vi "ParseObjectXML.vi"(8 "error in (no error)":errorcluster, 11 "Object XML":string="  <Object>\n    <Name>Blah</Name>\n    <Class>CoilQF_Test</Class>\n    <Config>\n      <NumElts>1</NumElts>\n      <String>\n        <Name>Rig_Location</Name>\n        <Val>Sydney</Val>\n      </String>\n    </Config>\n    <Validation>\n      <Method>\n        <Name>GetVersion</Name>\n        <Value>V1.2</Value>\n      </Method>\n      <Method>\n        <Name>GetCallChain</Name>\n        <Value>ViKingBase:Blah</Value>\n      </Method>\n    </Validation>\n    <Objects>\n          <Object>\n            <Name>Crud</Name>\n            <Class>Crud_class</Class>\n          </Object>\n      <Object>\n        <Name>QFM</Name>\n        <Class>QFM_T457232</Class>\n        <Config>\n          <NumElts>1</NumElts>\n          <String>\n            <Name>COM_Port</Name>\n            <Val>COM4</Val>\n          </String>\n        </Config>\n        <Validation>\n          <Method>\n            <Name>GetModel</Name>\n            <Value>T457635</Value>\n          </Method>\n          <Method>\n            <Name>GetSN</Name>\n            <Value>12</Value>\n          </Method>\n        </Validation>\n      </Object>\n    </Objects>\n    <Ancestors>\n      <Ancestor>\n        <Class>ViKing_Test_Base</Class>\n        <Config>\n          <NumElts>1</NumElts>\n          <String>\n            <Name>Rig_Location</Name>\n            <Val>Sydney</Val>\n          </String>\n        </Config>\n        <Objects>\n          <Object>\n            <Name>TestView</Name>\n            <Class>TestView_Tree</Class>\n          </Object>\n          <Object>\n            <Name>Crud</Name>\n            <Class>Crud_class</Class>\n          </Object>\n        </Objects>\n      </Ancestor>\n    </Ancestors>\n  </Object>") -> (0 "error out":errorcluster, 3 "Object Cluster":T1)   [LabVIEW 2022 SP3, in "ViPER.lvlib" / "ViPER.lvclass"]
doc: "### BSD License (http://www.opensource.org/licenses/bsd-license.php) Begin ###\n\nCopyright (c) 2018 Kurt Friday www.medulla.net\n\nAll rights reserved.\n\nRedistribution and use in source and binary forms, with or without\nmodification, are permitted provided that the following conditions are met:\n\n * Redistributions of source code must retain the above copyright\n notice, this list of conditions and the following disclaimer.\n\n * Redistributions in binary form must reproduce the above copyright\n notice, this list of conditions and the following disclaimer in the\n documentation and/or other materials provided with the distribution.\n\n * Neither the name of the <organization> nor the\n names of its contributors may be used to endorse or promote products\n derived from this software without specific prior written permission.\n\nTHIS SOFTWARE IS PROVIDED BY THE COPYRIGHT HOLDERS AND CONTRIBUTORS \"AS IS\" AND\nANY EXPRESS OR IMPLIED WARRANTIES, INCLUDING, BUT NOT LIMITED TO, THE IMPLIED\nWARRANTIES OF MERCHANTABILITY AND FITNESS FOR A PARTICULAR PURPOSE ARE\nDISCLAIMED. IN NO EVENT SHALL <COPYRIGHT HOLDER> BE LIABLE FOR ANY\nDIRECT, INDIRECT, INCIDENTAL, SPECIAL, EXEMPLARY, OR CONSEQUENTIAL DAMAGES\n(INCLUDING, BUT NOT LIMITED TO, PROCUREMENT OF SUBSTITUTE GOODS OR SERVICES;\nLOSS OF USE, DATA, OR PROFITS; OR BUSINESS INTERRUPTION) HOWEVER CAUSED AND\nON ANY THEORY OF LIABILITY, WHETHER IN CONTRACT, STRICT LIABILITY, OR TORT\n(INCLUDING NEGLIGENCE OR OTHERWISE) ARISING IN ANY WAY OUT OF THE USE OF THIS\nSOFTWARE, EVEN IF ADVISED OF THE POSSIBILITY OF SUCH DAMAGE."
uses:
  ViPER.lvclass
  ObjectDefinition.ctl
  Ancestor.ctl
  <vilib>/xml/Load XML String.vi
  <vilib>/xml/Close Reference(Node).vi
  <vilib>/xml/NI_XML.lvlib
panel:
  # "### BSD License (http://www.opensource.org/licenses/bsd-license.php) Begin ###\n\nCopyright (c) 2018  Kurt Friday www.medulla.net\n\nAll rights reserved.\n\nRedistribution and use in source and binary forms, with or without\nmodification, are permitted provided that the following conditions are met:\n\n    * Redistributions of source code must retain the above copyright\n      notice, this list of conditions and the following disclaimer.\n\n    * Redistributions in binary form must reproduce the above copyright\n      notice, this list of conditions and the following disclaimer in the\n      documentation and/or other materials provided with the distribution.\n\n    * Neither the name of the <organization> nor the\n      names of its contributors may be used to endorse or promote products\n      derived from this software without specific prior written permission.\n\nTHIS SOFTWARE IS PROVIDED BY THE COPYRIGHT HOLDERS AND CONTRIBUTORS \"AS IS\" AND\nANY EXPRESS OR IMPLIED WARRANTIES, INCLUDING, BUT NOT LIMITED TO, THE IMPLIED\nWARRANTIES OF MERCHANTABILITY AND FITNESS FOR A PARTICULAR PURPOSE ARE\nDISCLAIMED. IN NO EVENT SHALL <COPYRIGHT HOLDER> BE LIABLE FOR ANY\nDIRECT, INDIRECT, INCIDENTAL, SPECIAL, EXEMPLARY, OR CONSEQUENTIAL DAMAGES\n(INCLUDING, BUT NOT LIMITED TO, PROCUREMENT OF SUBSTITUTE GOODS OR SERVICES;\nLOSS OF USE, DATA, OR PROFITS; OR BUSINESS INTERRUPTION) HOWEVER CAUSED AND\nON ANY THEORY OF LIABILITY, WHETHER IN CONTRACT, STRICT LIABILITY, OR TORT\n(INCLUDING NEGLIGENCE OR OTHERWISE) ARISING IN ANY WAY OUT OF THE USE OF THIS\nSOFTWARE, EVEN IF ADVISED OF THE POSSIBILITY OF SUCH DAMAGE."
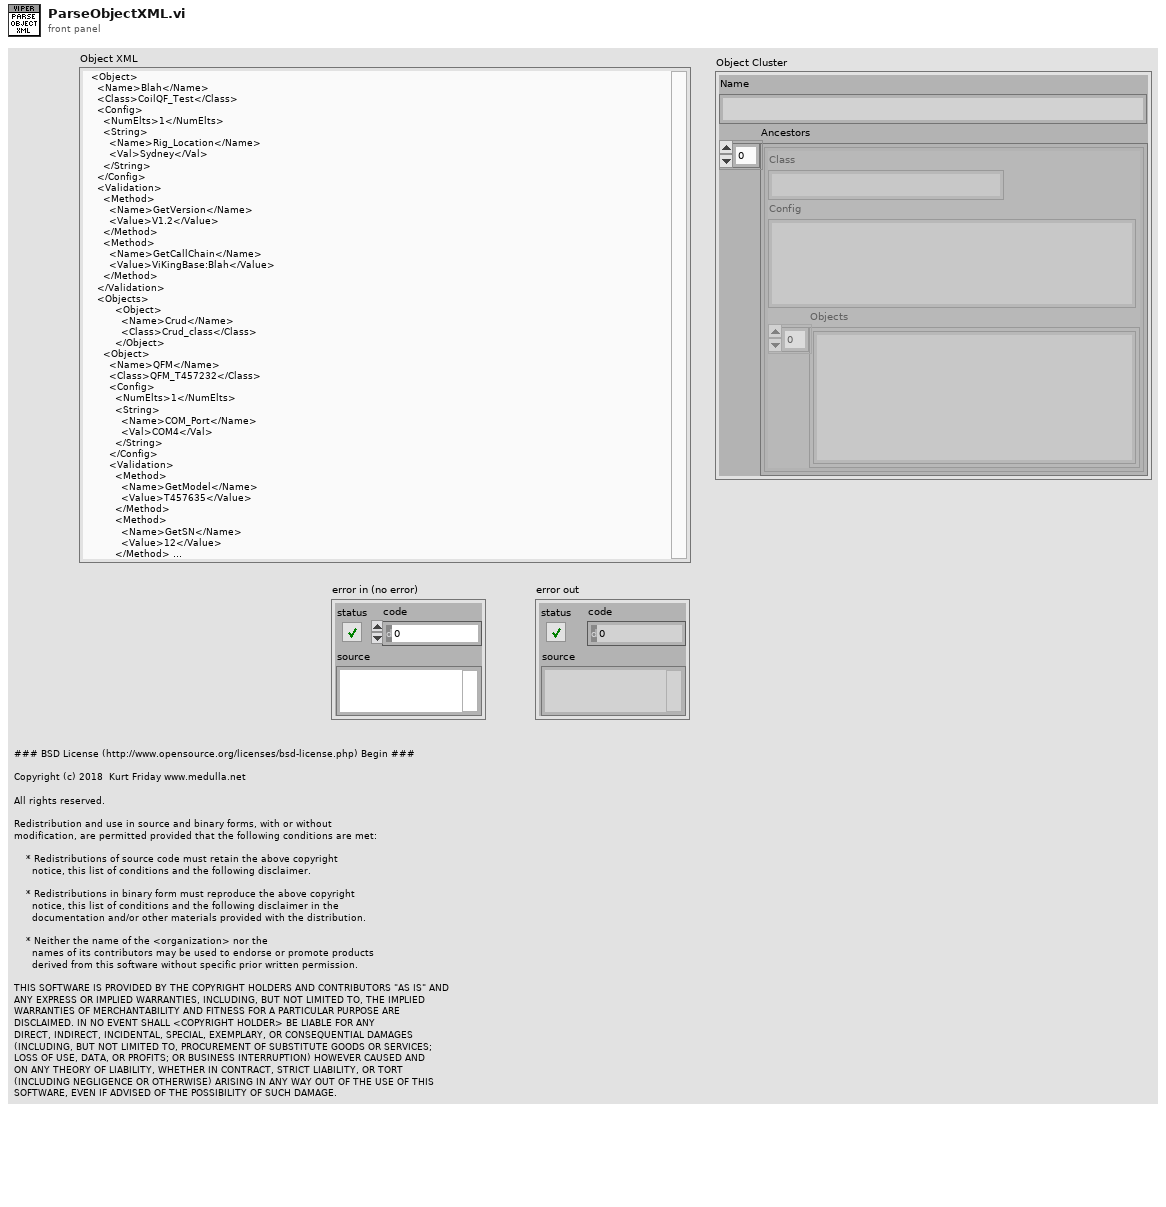
[diagram p1: front panel]
types:
  T1 = typedef "ViPER.lvlib/ViPER.lvclass/ObjectDefinition.ctl" = cluster{"Name":string, "Ancestors":T2[]}
  T2 = typedef "ViPER.lvlib/ViPER.lvclass/Ancestor.ctl" = cluster{"Class":string, "Config":string, "Objects":string[]}
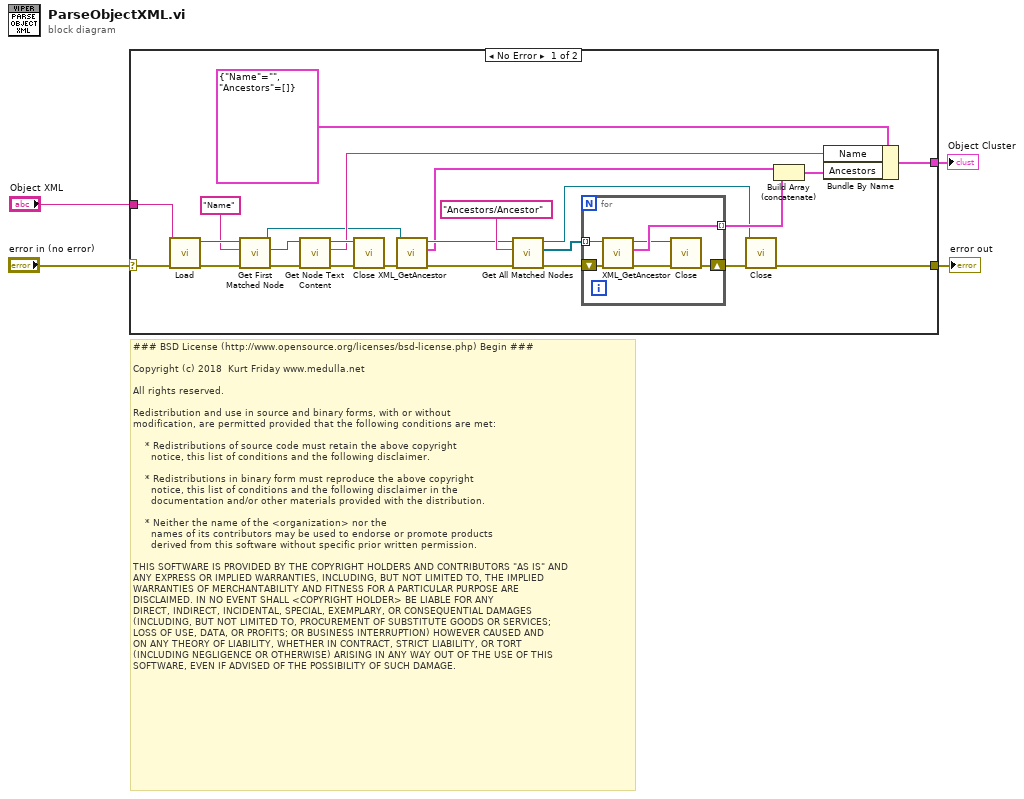
[diagram p0: block diagram]
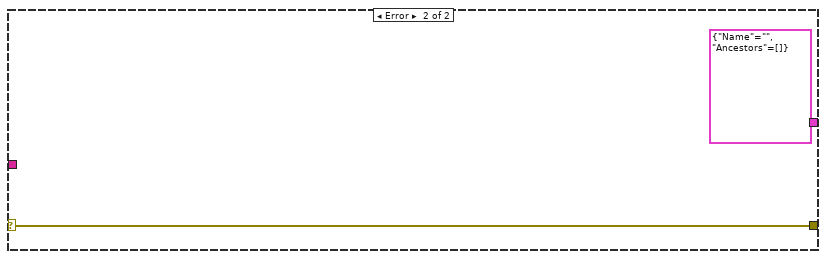
[diagram p2: hidden frame]
diagram:
  # "### BSD License (http://www.opensource.org/licenses/bsd-license.php) Begin ###\n\nCopyright (c) 2018  Kurt Friday www.medulla.net\n\nAll rights reserved.\n\nRedistribution and use in source and binary forms, with or without\nmodification, are permitted provided that the following conditions are met:\n\n    * Redistributions of source code must retain the above copyright\n      notice, this list of conditions and the following disclaimer.\n\n    * Redistributions in binary form must reproduce the above copyright\n      notice, this list of conditions and the following disclaimer in the\n      documentation and/or other materials provided with the distribution.\n\n    * Neither the name of the <organization> nor the\n      names of its contributors may be used to endorse or promote products\n      derived from this software without specific prior written permission.\n\nTHIS SOFTWARE IS PROVIDED BY THE COPYRIGHT HOLDERS AND CONTRIBUTORS \"AS IS\" AND\nANY EXPRESS OR IMPLIED WARRANTIES, INCLUDING, BUT NOT LIMITED TO, THE IMPLIED\nWARRANTIES OF MERCHANTABILITY AND FITNESS FOR A PARTICULAR PURPOSE ARE\nDISCLAIMED. IN NO EVENT SHALL <COPYRIGHT HOLDER> BE LIABLE FOR ANY\nDIRECT, INDIRECT, INCIDENTAL, SPECIAL, EXEMPLARY, OR CONSEQUENTIAL DAMAGES\n(INCLUDING, BUT NOT LIMITED TO, PROCUREMENT OF SUBSTITUTE GOODS OR SERVICES;\nLOSS OF USE, DATA, OR PROFITS; OR BUSINESS INTERRUPTION) HOWEVER CAUSED AND\nON ANY THEORY OF LIABILITY, WHETHER IN CONTRACT, STRICT LIABILITY, OR TORT\n(INCLUDING NEGLIGENCE OR OTHERWISE) ARISING IN ANY WAY OUT OF THE USE OF THIS\nSOFTWARE, EVEN IF ADVISED OF THE POSSIBILITY OF SUCH DAMAGE."
  n1 = case shown="No Error" "error in (no error)" {
    selector: "error in (no error)" -> [w5 w37]
    tunnel: "Object XML" -> [w28 _]
    tunnel: [w7 T1 {"Name"="", "Ancestors"=[]} ("Object")] -> w3
    tunnel: [w6 w37] -> w2
    frame No Error {
      n2 = call-poly <vilib>:"Load.vi"("XML string"=w28, "error in (no error)"=w5) -> ("DOM document out"=w27:refnum<k20>, "error out"=w29:errorcluster)  [unwired: 11 in, 1 out]
      n3 = call <vilib>:"Get First Matched Node.vi"("error in (no error)"=w29, "XPath expression"="Name", "node in"=w27) -> ("error out"=w24:errorcluster, "node result"=w21:refnum<k20>, "node out"=w18:refnum<k20>)  [unwired: 6 in]
      n4 = call <vilib>:"Get Node Text Content.vi"("error in (no error)"=w24, "node in"=w21) -> ("error out"=w23:errorcluster, "node text"=w20:string, "node out"=w22:refnum<k20>)  [unwired: 7 in]
      n5 = call-poly <vilib>:"Close.vi"("error in (no error)"=w23, "node"=w22) -> ("error out"=w19:errorcluster)  [unwired: 7 out]
      n6 = call "XML_GetAncestor.vi"("error in (no error)"=w19, "node in"=w18) -> ("error out"=w16:errorcluster, "output cluster"=w12:T2, "node out"=w15:refnum<k20>)  [unwired: 7 in]
      n7 = call <vilib>:"Get All Matched Nodes.vi"("error in (no error)"=w16, "XPath expression"="Ancestors/Ancestor", "node in"=w15) -> ("error out"=w13:errorcluster, "node result array"=w14:refnum<k20>[], "node out"=w8:refnum<k20>)  [unwired: 6 in]
      n8 = for {
        tunnel: w14 -> [w34] mode=indexing
        shift-right: [w31] -> w9
        shift-left: w13 -> [w35]
        tunnel: [w33] -> w11 mode=indexing
        n9 = call "XML_GetAncestor.vi"("error in (no error)"=w35, "node in"=w34) -> ("error out"=w32:errorcluster, "output cluster"=w33:T2, "node out"=w30:refnum<k20>)  [unwired: 7 in]
        n10 = call-poly <vilib>:"Close.vi"("error in (no error)"=w32, "node"=w30) -> ("error out"=w31:errorcluster)  [unwired: 7 out]
      }
      n11 = call-poly <vilib>:"Close.vi"("error in (no error)"=w9, "node"=w8) -> ("error out"=w6:errorcluster)  [unwired: 7 out]
      n12 = Build Array (concatenate)(w12, w11) -> (w10:T2[])
      n13 = Bundle By Name(cluster=T1 {"Name"="", "Ancestors"=[]} ("Object"), "Name"=w20, "Ancestors"=w10) -> (w7:T1)
    }
    frame Error {
    }
  }
  "Object Cluster" <- w3
  "error out" <- w2
